vi "PH_Beamline.get BB State.vi"(0 "i ref in":refnum<vi>, 2 "Black Box Instance":T1="PA_CH1_BB", 5 "error in (no error)":errorcluster) -> (14 "i ref out":refnum<vi>, 15 "off/false/out?":bool, 16 "on/true/in?":bool, 17 "Black Box State":T2 items=["no info", "off/false/out", "on/true/in", "Failure", "Alarm", "Status 1", "Status 2", "Status 3"], 18 "off/false/out or on/true/in?":bool, 19 "error out":errorcluster)   [LabVIEW 2009]
doc: "This VI gets the state of the selected BLACK BOX."
uses:
  PH_Beamline.lvlib
  CSUser/DIMServiceTools/Status.ctl
  PH_Beamline.Black Box Instances.ctl
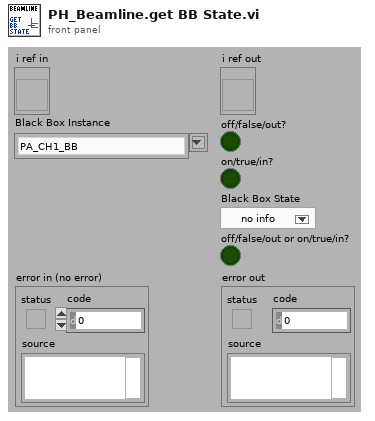
[diagram p1: front panel]
types:
  T1 = typedef "PH_Beamline.lvlib/PH_Beamline.Black Box Instances.ctl" = string
  T2 = typedef "Status.ctl" = i16
  T3 = typedef "PH_Beamline.lvlib/PH_Beamline.i attribute.ctl" = cluster{"GUI Refs":cluster{"PA ok":refnum<vi>, "MA ok":refnum<vi>, "fs FE ok":refnum<vi>, "ns FE ok":refnum<vi>, "PA ED ok":refnum<vi>, "MAS ok":refnum<vi>, "Booster ok":refnum<vi>, "Mirrortower ok":refnum<vi>, "In.-Box ok":refnum<vi>, "Compressor ok":refnum<vi>, "Experiment LB ok":refnum<vi>, "Experiment LL ok":refnum<vi>, "PHELIX_Beckhoff_Watchdog":refnum<vi>, "Shutters closed":refnum<vi>}, "Refs BL MA":refnum<vi>[], "Refs BL MA-IB":refnum<vi>[], "Refs BL fs":refnum<vi>[], "Refs BL PA ED":refnum<vi>[], "Refs BL MAS":refnum<vi>[], "Refs BL Boo":refnum<vi>[], "Refs BL ns":refnum<vi>[], "Refs BL Mirrortower":refnum<vi>[], "Refs BL Compressor":refnum<vi>[], "Refs BL Exp LB":refnum<vi>[], "Radiation Safety":cluster{"Exp Laserbay":cluster{"Ref Op Mode":refnum<vi>, "Ref Laserbay evacuated":refnum<vi>, "Tagname LB evacuated":string, "Shot Mode":T4, "Laserbay evacuated?":i32, "Tagname HV room locked":string, "HV room locked?":i32, "Ref HV room locked":refnum<vi>, "Tagname bridged?":string, "Ref Bridge":refnum<vi>, "I<1E18W/cm²":bool}, "Exp Laserlab":cluster{"Ref Op Mode":refnum<vi>, "Ref Laserlab evacuated":refnum<vi>, "Tagname LL evacuated":string, "Shot Mode":T4, "Laserlab evacuated?":i32, "Tagname bridged?":string, "Ref Bridge":refnum<vi>, "I<1E18W/cm²":bool}}, "Refs BL LL":refnum<vi>[], "PP Igni Heating GUI Refs":refnum<vi>[], "PP Igni Heating Tagnames ":string[], "Refs BL PA":cluster{"undelayed Line before Shutter":refnum<vi>[], "undelayed Line after Shutter":refnum<vi>[], "before Bypass":refnum<vi>[], "delayed Line before Shutter":refnum<vi>[], "delayed Line after Shutter":refnum<vi>[], "before Shutter Input":refnum<vi>[], "after Shutter Input":refnum<vi>[], "Bypass":refnum<vi>[], "before Shutter Exit":refnum<vi>[], "after Shutter Exit":refnum<vi>[], "to MA":refnum<vi>[], "to Lab":refnum<vi>[]}, "Service ID":cluster{"YLF_BL_Status":i32, "fs_BL_Status":i32, "fs_YLF_BL_Status":i32, "ns_BL_Status":i32, "PA_Input_BL_Status":i32, "PA_UnDelay_BL_Status":i32, "PA_Delay_BL_Status":i32, "PA_BL_Status":i32, "PA_Bypass_BL_Status":i32, "PA_Exit_BL_Status":i32, "PA_LL_BL_Status":i32, "LL_BL_Status":i32, "PA_MA_BL_Status":i32, "MA_Exit_BL_Status":i32, "MA_Z6_BL_Status":i32, "Z6_BL_Status":i32, "MA_LB_BL_Status":i32, "LB_TB2_BL_Status":i32, "PA_before_Bypass_BL_Status":i32, "LB_TB3_BL_Status":i32}, "BL":cluster{"YLF_BL_Status":i32, "fs_BL_Status":i32, "fs_YLF_BL_Status":i32, "ns_BL_Status":i32, "PA_Input_BL_Status":i32, "PA_UnDelay_BL_Status":i32, "PA_Delay_BL_Status":i32, "PA_BL_Status":i32, "PA_Bypass_BL_Status":i32, "PA_Exit_BL_Status":i32, "PA_LL_BL_Status":i32, "LL_BL_Status":i32, "PA_MA_BL_Status":i32, "MA_Exit_BL_Status":i32, "MA_Z6_BL_Status":i32, "Z6_BL_Status":i32, "MA_LB_BL_Status":i32, "LB_TB2_BL_Status":i32, "PA_before_Bypass_BL_Status":i32, "LB_TB3_BL_Status":i32}, "State Subsystems":cluster{"PA":bool, "MA":bool, "ns FE":bool, "fs FE":bool, "PA ED":bool, "In.-Box":bool, "MAS":bool, "Booster":bool, "Mirrortower":bool, "Compressor":bool, "Experiment LB":bool, "Experiment LL":bool}}
  T4 = typedef "Operation Mode.ctl" = i32
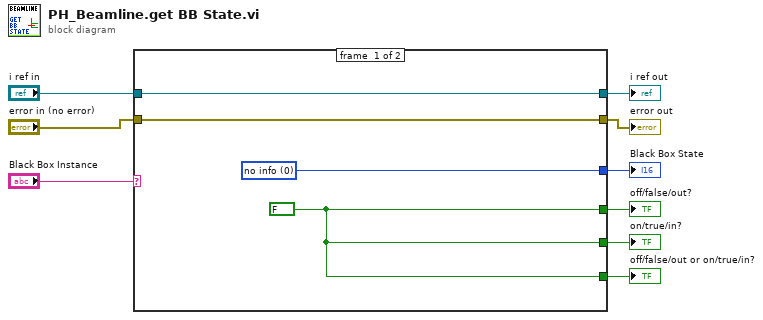
[diagram p0: block diagram]
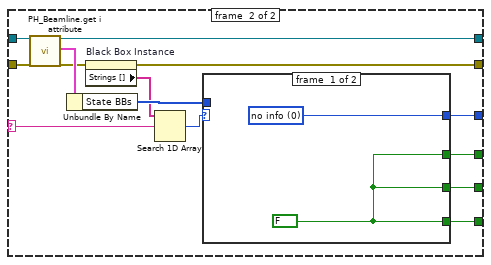
[diagram p2: hidden frame]
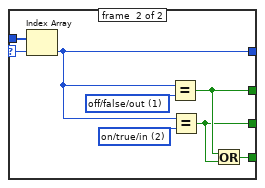
[diagram p3: hidden frame]
diagram:
  n1 = case shown="Default" "Black Box Instance" {
    selector: "Black Box Instance" -> [_ w18]
    tunnel: "error in (no error)" -> [w12 w26]
    tunnel: "i ref in" -> [w13 w25]
    tunnel: [w13 w24] -> w7
    tunnel: [w11 w23] -> w6
    tunnel: [w12 w19] -> w5
    tunnel: [w10 w16] -> w3
    tunnel: [w10 w15] -> w2
    tunnel: [w10 w14] -> w1
    frame #0 {
      w11 = T2 0 items=["no info", "off/false/out", "on/true/in", "Failure", "Alarm", "Status 1", "Status 2", "Status 3"] ("State")
      w10 = FALSE
    }
    frame #1 {
      n2 = call "PH_Beamline.get i attribute.vi"("i ref in"=w25, "error in (no error)"=w26) -> ("i ref out"=w24:refnum<vi>, "i attribute"=w27:T3, "error out"=w20:errorcluster)  [unwired: 15 in]
      n3 = Unbundle By Name(w27) -> ("State BBs"=w22:T2[])
      n4 = property on="Black Box Instance" class="ComboBox"(error in=w20) -> (error out=w19:errorcluster, "Strings []"=w21:string[])  [unwired: 1 in, 1 out]
      n5 = Search 1D Array(1D array=w21, element=w18) -> (index of element=w17:i32)  [unwired: 1 in]
      n6 = case shown="Default" w17 {
        selector: w17 -> [_ w36]
        tunnel: [w29 w34] -> w23
        tunnel: w22 -> [_ w37]
        tunnel: [w28 w32] -> w16
        tunnel: [w28 w31] -> w15
        tunnel: [w28 w30] -> w14
        frame #0 {
          w28 = FALSE
          w29 = T2 0 items=["no info", "off/false/out", "on/true/in", "Failure", "Alarm", "Status 1", "Status 2", "Status 3"] ("State")
        }
        frame #1 {
          w33 = T2 2 items=["no info", "off/false/out", "on/true/in", "Failure", "Alarm", "Status 1", "Status 2", "Status 3"] ("y")
          w35 = T2 1 items=["no info", "off/false/out", "on/true/in", "Failure", "Alarm", "Status 1", "Status 2", "Status 3"] ("y")
          n7 = Index Array(array=w37, index=w36) -> (element=w34:T2)
          n8 = Equal?(x=w34, y=w35) -> (x = y?=w32:bool)
          n9 = Equal?(x=w34, y=w33) -> (x = y?=w31:bool)
          n10 = Or(x=w32, y=w31) -> (x .or. y?=w30:bool)
        }
      }
    }
  }
  "i ref out" <- w7
  "error out" <- w5
  "Black Box State" <- w6
  "off/false/out?" <- w3
  "on/true/in?" <- w2
  "off/false/out or on/true/in?" <- w1
